vi "Init.vi"(5 "Bus In":refnum<class "Bus.lvclass">, 7 "Cluster":T1, 8 "error in (no error)":errorcluster, 9 "Init or Array":bool, 10 "Array":dbl[](array[numeric]), 11 "Single Channel in":refnum<class "Single Channel.lvclass">) -> (0 "error out":errorcluster, 2 "Bus Out":refnum<class "Bus.lvclass">, 3 "Single Channel out":refnum<class "Single Channel.lvclass">)   [LabVIEW 2024, in "Single Channel.lvclass"]
uses:
  Single Channel.lvclass
  Scaling/Scaling.lvclass
  Bus/Bus.lvclass
  Single Channel.lvclass/Single Channel.ctl
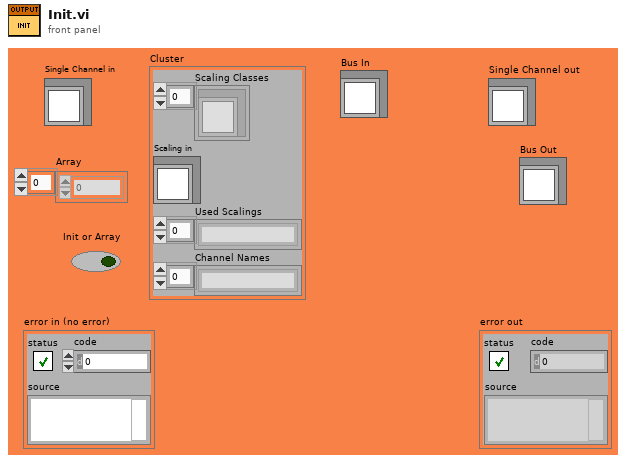
[diagram p1: front panel]
types:
  T1 = cluster{"Scaling Classes":refnum<class "Scaling.lvclass">[], "Scaling in":refnum<class "Scaling.lvclass">, "Used Scalings":string[], "Channel Names":string[]}
  T2 = cluster{"Parsing String":string, "Channel Name":string, "Enabled":bool, "Initial Value":dbl}[]
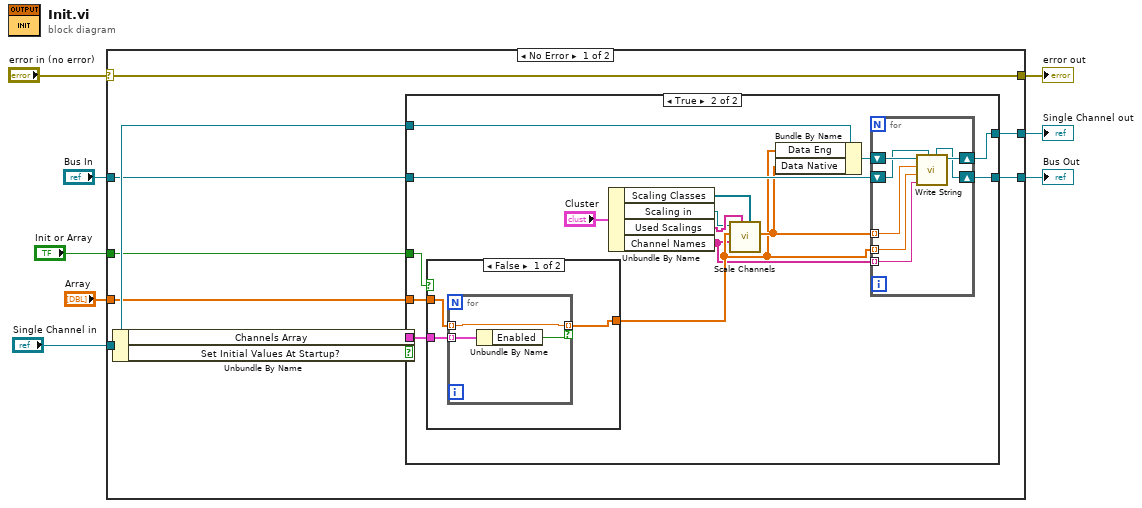
[diagram p0: block diagram]
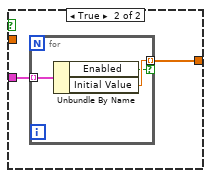
[diagram p3: hidden frame]
diagram:
  n1 = case shown="No Error" "error in (no error)" {
    selector: "error in (no error)" -> [w17 w54]
    tunnel: [w17 w54] -> w7
    tunnel: [w12 w55] -> w6
    tunnel: "Single Channel in" -> [w16 w55]
    tunnel: "Init or Array" -> [w15 _]
    tunnel: "Array" -> [w13 _]
    tunnel: "Bus In" -> [w11 w53]
    tunnel: [w10 w53] -> w1
    frame No Error {
      n2 = Unbundle By Name(w16) -> ("Channels Array"=w14:T2, "Set Initial Values At Startup?"=w9:bool)
      n3 = case shown="True" w9 {
        tunnel: w16 -> [w19 w34]
        tunnel: w15 -> [_ w33]
        tunnel: w14 -> [_ w32]
        tunnel: w13 -> [_ w31]
        tunnel: [w19 w25] -> w12
        tunnel: w11 -> [w18 w24]
        tunnel: [w18 w23] -> w10
        frame False {
        }
        frame True {
          n4 = case shown="False" w33 {
            tunnel: w32 -> [w44 w49]
            tunnel: [w43 w48] -> w21
            tunnel: w31 -> [w42 _]
            frame False {
              n5 = for {
                tunnel: w44 -> [w47] mode=indexing
                tunnel: [w46] -> w43 mode=indexing if=w45
                tunnel: w42 -> [w46] mode=indexing
                n6 = Unbundle By Name(w47) -> ("Enabled"=w45:bool)
              }
            }
            frame True {
              n7 = for {
                tunnel: w49 -> [w52] mode=indexing
                tunnel: [w51] -> w48 mode=indexing if=w50
                n8 = Unbundle By Name(w52) -> ("Enabled"=w50:bool, "Initial Value"=w51:dbl)
              }
            }
          }
          n9 = Unbundle By Name("Cluster") -> ("Scaling Classes"=w28:refnum<class "Scaling.lvclass">[], "Scaling in"=w29:refnum<class "Scaling.lvclass">, "Used Scalings"=w30:string[], "Channel Names"=w20:string[])
          n10 = call "Scale Channels.vi"("Scaling Classes"=w28, "Used Scalings"=w30, "Channel Names"=w20, "Values In"=w21, "Scaling in"=w29) -> ("Values Out"=w22:dbl[])  [unwired: 4 in, 2 out]
          n11 = Bundle By Name(cluster=w34, "Data Eng"=w21, "Data Native"=w22) -> (w26:refnum<class "Single Channel.lvclass">)
          n12 = for {
            tunnel: w22 -> [w37] mode=indexing
            tunnel: w21 -> [w36] mode=indexing
            tunnel: w20 -> [w35] mode=indexing
            shift-right: [w40] -> w25
            shift-left: w26 -> [w41]
            shift-right: [w38] -> w23
            shift-left: w24 -> [w39]
            n13 = call-dynamic "Write String.vi"("Bus In"=w39, "Channel Name"=w35, "Data Value Engineering"=w36, "Data Value Native"=w37, "NI Digital in"=w41) -> ("NI Digital out"=w40:refnum<class "Single Channel.lvclass">, "Bus Out"=w38:refnum<class "Bus.lvclass">)  [unwired: 4 in, 1 out]
          }
        }
      }
    }
    frame Error {
    }
  }
  "error out" <- w7
  "Single Channel out" <- w6
  "Bus Out" <- w1
